vi "Teleop.vi"(10 "Match Info":T1={"Autonomous Elapsed Seconds"=0.0, "TeleOp Elapsed Seconds"=0.0, "Disabled Elapsed Seconds"=0.0, "Visited Autonomous"=FALSE, "Visited TeleOp"=FALSE, "Visited Disabled"=FALSE, "Autonomous Settings"={"Autonomous Style"=enum."Independent", "VI Refnum"=refnum}}, 11 "Call Context":T2) -> ()   [LabVIEW 2013]
doc: "This VI is called for each TeleOp packet received from the DS where the robot is not disabled. It is often used to read from the joysticks and update I/O or to update setpoints for timed control loops. It should complete and return within 20 milliseconds or it may miss DS packets."
uses:
  <vilib>/Rock Robotics/WPI/DriverStation/WPI_DriverStationDerivedRobotMode.ctl
  <vilib>/Rock Robotics/WPI/DriverStation/WPI_DriverStationMatch Info.ctl
  <vilib>/Rock Robotics/WPI/DriverStation/DriverStationLCD/WPI_DriverStationLCDLCDLine.ctl
  Robot Global Data.vi
  <vilib>/Rock Robotics/WPI/Joystick/WPI_JoystickGetSetRefNum.vi
  <vilib>/Rock Robotics/WPI/RobotDrive/WPI_RobotDriveGetSetRefNum.vi
  <vilib>/Rock Robotics/WPI/Solenoid/WPI_SolenoidSetEnum.vi
  <vilib>/Rock Robotics/WPI/Solenoid/WPI_SolenoidValue.ctl
panel:
  out "Numeric 1":dbl(slide) scale=0.0..100.0
  out "Boolean 2":bool
  out "Boolean 1":bool
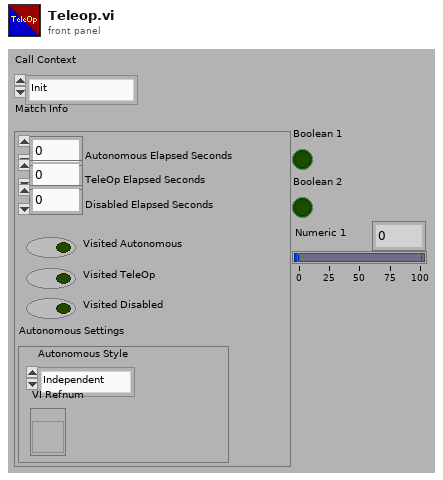
[diagram p1: front panel]
types:
  T1 = typedef "WPI_DriverStationMatch Info.ctl" = cluster{"Autonomous Elapsed Seconds":dbl, "TeleOp Elapsed Seconds":dbl, "Disabled Elapsed Seconds":dbl, "Visited Autonomous":bool, "Visited TeleOp":bool, "Visited Disabled":bool, "Autonomous Settings":cluster{"Autonomous Style":enum16{"Iterative", "Independent"}, "VI Refnum":refnum<vi>}}
  T2 = typedef "WPI_DriverStationDerivedRobotMode.ctl" = enum16{"Init", "Execute", "Stop"}
  T3 = typedef "WPI_DriverStationLCDLCDLine.ctl" = enum16{"Main - Line 1", "User - Line 2", "User - Line 3", "User - Line 4", "User - Line 5", "User - Line 6"}
  T4 = typedef "WPI_JoystickDevRef.ctl" = cluster{"Device":T5}
  T5 = typedef "WPI_JoystickDeviceEnum.ctl" = enum16{"USB 1", "USB 2", "USB 3", "USB 4", "Kinect 1", "Kinect 2"}
  T6 = typedef "WPI_JoystickButtonState.ctl" = cluster{"Button 1":bool, "Button 2":bool, "Button 3":bool, "Button 4":bool, "Button 5":bool, "Button 6":bool, "Button 7":bool, "Button 8":bool, "Button 9":bool, "Button 10":bool, "Button 11":bool, "Button 12":bool}
  T7 = cluster{"axis 1 (x)":dbl, "axis 2 (y)":dbl, "axis 3 (throttle)":dbl, "axis 4":dbl, "axis 5":dbl, "axis 6":dbl}
  T8 = typedef "WPI_SolenoidValue.ctl" = enum16{"Off", "On", "Forward", "Reverse"}
  T9 = typedef "WPI_SolenoidDevRef.ctl" = cluster{"DevStatus":errorcluster, "Solenoid Module":T10, "Forward Solenoid Channel":T11, "Reverse Solenoid Channel":T11}
  T10 = typedef "FPGA_TypedefSolenoidModule.ctl" = enum16{"Solenoid Module 1", "Solenoid Module 2"}
  T11 = typedef "WPI_SolenoidChannel.ctl" = enum8{"Solenoid 1", "Solenoid 2", "Solenoid 3", "Solenoid 4", "Solenoid 5", "Solenoid 6", "Solenoid 7", "Solenoid 8", "Invalid"}
  T12 = typedef "WPI_RobotDriveDevRef.ctl" = cluster{"DevStatus":errorcluster, "Motors[]":T13[], "Square Inputs":bool, "Max Output":dbl, "Isochronous":bool}
  T13 = typedef "WPI_MotorControlDeviceRef.ctl" = cluster{"DeviceStatus":errorcluster, "Type":enum16{"PWM", "CAN"}, "PWM":cluster{"Digital Module":T14, "PWM Channel":T15, "DeadBand":T16}, "CAN":cluster{"Device Number":u8, "Control Mode":T17, "Semaphore":T18, "Max Vout":dbl}, "Invert":bool, "TransformRef":T19, "InvTransformRef":T19}
  T14 = typedef "FPGA_TypedefDigitalModule.ctl" = enum16{"Digital Module 1", "Digital Module 2"}
  T15 = typedef "FPGA_DIOPWMChannel.ctl" = enum8{"PWM 1", "PWM 2", "PWM 3", "PWM 4", "PWM 5", "PWM 6", "PWM 7", "PWM 8", "PWM 9", "PWM 10", "Invalid"}
  T16 = typedef "WPI_PWMDeadband.ctl" = cluster{"Name":string, "maxPositivePwm":i32, "minPositivePwm":i32, "centerPwm":i32, "maxNegativePwm":i32, "minNegativePwm":i32, "angularRange":u16}
  T17 = typedef "WPI_CANJaguar_ControlMode.ctl" = enum8{"Percent VBus", "Current", "Speed", "Position", "Voltage"}
  T18 = typedef "Semaphore RefNum" = refnum<k1>
  T19 = typedef "WPI_PWMTransform_ConPane.ctl" = refnum<vi>
  T20 = enum16{"Start", "Reset", "Reset 2", "Reset Delay", "Reset 3", "Manual", "Wait for Firing Latch", "Get ready to Fire", "Disengage Gearbox", "Ready to Fire", "Firing", "Firing Completed", "Reengage Gearbox"}
  T21 = typedef "WPI_DigitalInputDevRef.ctl" = cluster{"DevStatus":errorcluster, "DIO Channel":T22, "Digital Module":T14}
  T22 = typedef "FPGA_DIOChannel.ctl" = enum8{"DIO 1", "DIO 2", "DIO 3", "DIO 4", "DIO 5", "DIO 6", "DIO 7", "DIO 8", "DIO 9", "DIO 10", "DIO 11", "DIO 12", "DIO 13", "DIO 14", "Invalid"}
  T23 = typedef "WPI_ServoDeviceRef.ctl" = cluster{"DeviceStatus":errorcluster, "Digital Module":T14, "PWM Channel":T15, "DeadBand":T16}
  T24 = typedef "WPI_AnalogChannelDevRef.ctl" = cluster{"DevStatus":errorcluster, "Analog Module":T25, "Analog Channel":T26}
  T25 = typedef "FPGA_TypedefAnalogModule.ctl" = enum16{"Analog Module 1", "Analog Module 2"}
  T26 = typedef "FPGA_AIChannel.ctl" = enum8{"AI 1", "AI 2", "AI 3", "AI 4", "AI 5", "AI 6", "AI 7", "AI 8", "Invalid"}
  T27 = typedef "WPI_RelayDevRef.ctl" = cluster{"DevStatus":errorcluster, "Relay Channel":T28, "Digital Module":T14, "Relay Direction":T29}
  T28 = typedef "FPGA_DIORelayChannel.ctl" = enum8{"Relay 1", "Relay 2", "Relay 3", "Relay 4", "Relay 5", "Relay 6", "Relay 7", "Relay 8", "Invalid"}
  T29 = typedef "WPI_RelayDirection.ctl" = enum16{"Both directions", "Forward only", "Reverse only"}
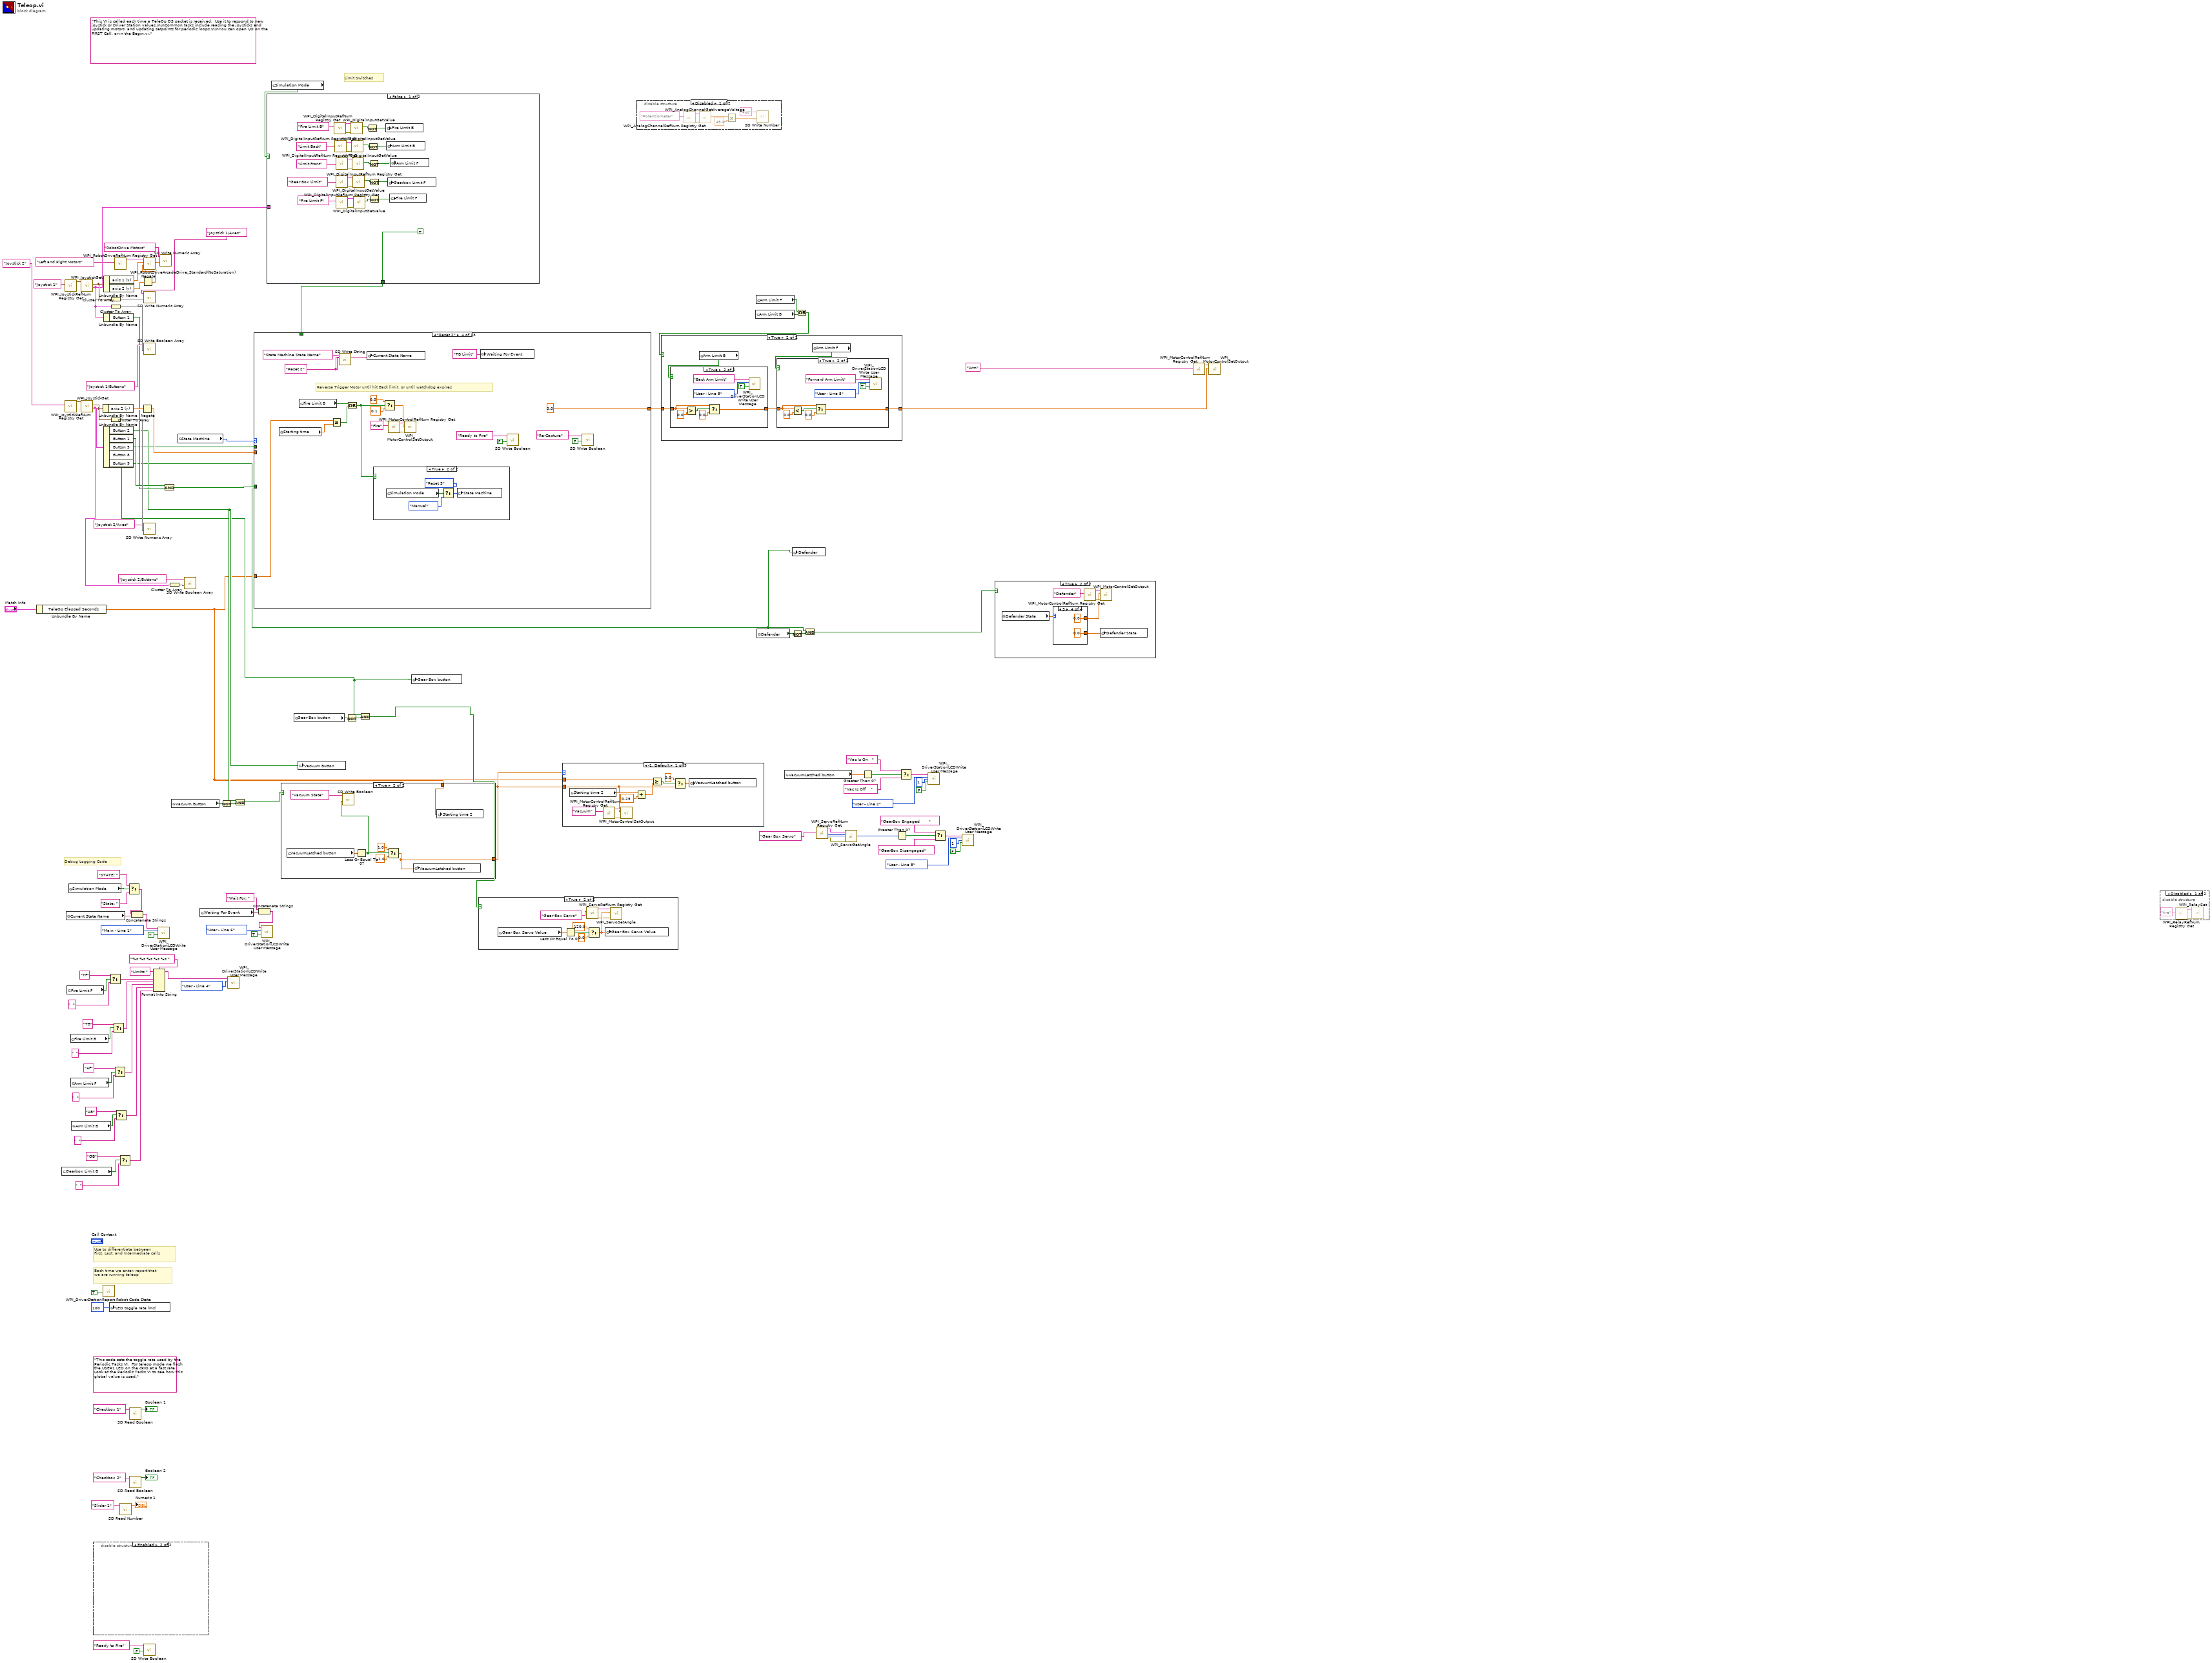
[diagram p0: block diagram]
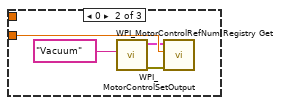
[diagram p2: hidden frame]
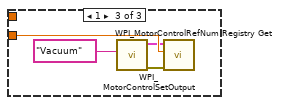
[diagram p3: hidden frame]
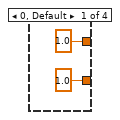
[diagram p6: hidden frame]
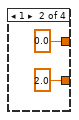
[diagram p7: hidden frame]
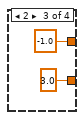
[diagram p8: hidden frame]
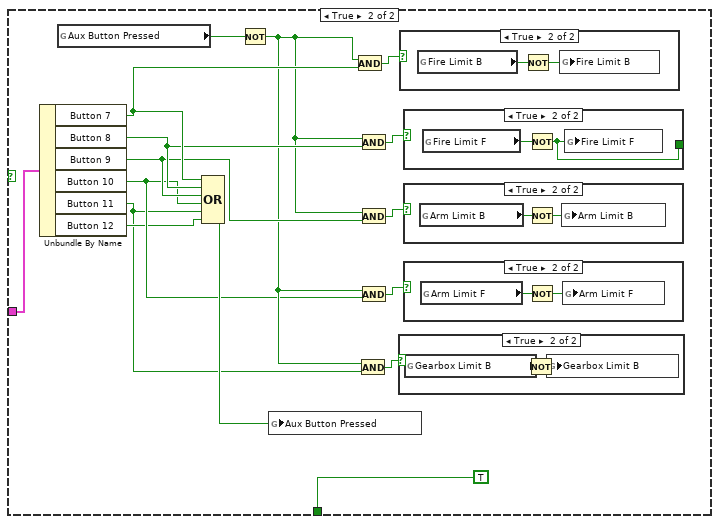
[diagram p9: hidden frame]
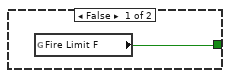
[diagram p13: hidden frame]
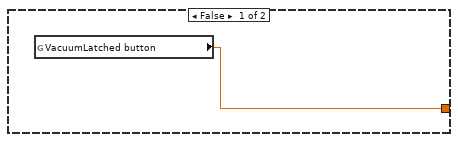
[diagram p15: hidden frame]
diagram:
  (unwired) "This code sets the toggle rate used by the Periodic Tasks VI.  For teleop mode we flash the USER1 LED on the cRIO at a fast rate.  Look at the Periodic Tasks VI to see how this global value is used."
  (unwired) "This VI is called each time a TeleOp DS packet is received.  Use it to respond to new joystick or Driver Station values.\n\nCommon tasks include reading the joysticks and updating motors, and updating setpoints for periodic loops.\n\nYou can open I/O on the FIRST Call, or in the Begin.vi."
  # "Limit Switches"
  # "Debug Logging Code"
  # "Each time we enter, report that\nwe are running teleop"
  # "Use to differentiate between\nFirst, Last, and Intermediate calls"
  n1 = Unbundle By Name("Match Info") -> ("TeleOp Elapsed Seconds"=w1:dbl)
  n2 = global read "Robot Global Data.vi" "Gearbox Limit B"() -> (w36:bool)
  n3 = call <vilib>:"WPI_JoystickRefNum Registry Get.vi"("refnum name"="Joystick 1") -> ("JoystickDevRef"=w115:T4)  [unwired: 1 in, 9 out]
  n4 = call <vilib>:"WPI_JoystickRefNum Registry Get.vi"("refnum name"="Joystick 2") -> ("JoystickDevRef"=w98:T4)  [unwired: 1 in, 9 out]
  n5 = global read "Robot Global Data.vi" "Current State Name"() -> (w63:string)
  n6 = global read "Robot Global Data.vi" "Fire Limit F"() -> (w40:bool)
  n7 = global read "Robot Global Data.vi" "Simulation Mode"() -> (w29:bool)
  n8 = global read "Robot Global Data.vi" "Fire Limit B"() -> (w39:bool)
  n9 = global read "Robot Global Data.vi" "Arm Limit F"() -> (w38:bool)
  n10 = global read "Robot Global Data.vi" "Arm Limit B"() -> (w37:bool)
  n11 = call <vilib>:"WPI_JoystickGet.vi"("JoystickDevRef"=w115) -> ("Buttons"=w25:T6, "Axes"=w110:T7)  [unwired: 1 in, 4 out]
  n12 = call <vilib>:"WPI_JoystickGet.vi"("JoystickDevRef"=w98) -> ("Buttons"=w92:T6, "Axes"=w95:T7)  [unwired: 1 in, 4 out]
  n13 = disable-structure shown="Enabled" {
    frame Disabled {
      n14 = case shown="True" {
        selector: _ -> [_ _]
        frame False {
          n15 = call <vilib>:"WPI_SolenoidRefNum Registry Get.vi"("refnum name"="Gear Box Clutch") -> ("error out"=w126:errorcluster, "SolenoidDevRef"=w127:T9)  [unwired: 9 in]
          n16 = call-poly <vilib>:"WPI_SolenoidSet.vi"("error in (no error)"=w126, "Value"=WPI_SolenoidValue."Off", "SolenoidDevRef"=w127) -> ()  [unwired: 7 in, 2 out]
          n17 = call <vilib>:"WPI_DriverStationLCDWrite User Message.vi"("line text"="Gear Box Clutch off", "line"=WPI_DriverStationLCDLCDLine."User - Line 2", "starting column"=i8 1, "clear line before write (T)"=FALSE) -> ()  [unwired: 11 in, 1 out]
        }
        frame True {
          n18 = call <vilib>:"WPI_SolenoidRefNum Registry Get.vi"("refnum name"="Gear Box Clutch") -> ("error out"=w134:errorcluster, "SolenoidDevRef"=w135:T9)  [unwired: 9 in]
          n19 = call-poly <vilib>:"WPI_SolenoidSet.vi"("error in (no error)"=w134, "Value"=WPI_SolenoidValue."Forward", "SolenoidDevRef"=w135) -> ()  [unwired: 7 in, 2 out]
          n20 = call <vilib>:"WPI_DriverStationLCDWrite User Message.vi"("line text"="Gear Box Clutch off", "line"=WPI_DriverStationLCDLCDLine."User - Line 2", "starting column"=i8 1, "clear line before write (T)"=FALSE) -> ()  [unwired: 11 in, 1 out]
        }
      }
    }
    frame Enabled {
    }
  }
  n21 = Unbundle By Name(w95) -> ("axis 2 (y)"=w91:dbl)
  n22 = call <vilib>:"WPI_DriverStationReport Robot Code State.vi"("TeleOp"=TRUE ("Autonomous")) -> ()  [unwired: 10 in, 1 out]
  n23 = Unbundle By Name(w110) -> ("axis 1 (x)"=w117:dbl, "axis 2 (y)"=w58:dbl)
  n24 = Unbundle By Name(w25) -> ("Button 1"=w89:bool)
  n25 = Unbundle By Name(w92) -> ("Button 2"=w80:bool, "Button 1"=w90:bool, "Button 5"=w66:bool, "Button 8"=w19:bool, "Button 9"=w18:bool)
  n26 = Select(t="TF", s=w40, f="  ") -> (s? t:f=w46:string)
  n27 = global write "Robot Global Data.vi" "LED toggle rate (ms)"(u32 100 ("LED ms toggle rate")) -> ()
  n28 = Cluster To Array(cluster=w110) -> (array=w109:dbl[])
  n29 = Cluster To Array(cluster=w25) -> (array=w112:bool[])
  n30 = Cluster To Array(cluster=w95) -> (array=w94:dbl[])
  n31 = Select(t="TB", s=w39, f="  ") -> (s? t:f=w45:string)
  n32 = Select(t="AF", s=w38, f="  ") -> (s? t:f=w44:string)
  n33 = call <vilib>:"WPI_RobotDriveRefNum Registry Get.vi"("refnum name"="Left and Right Motors") -> ("RobotDriveDevRef"=w118:T12)  [unwired: 1 in, 9 out]
  n34 = Select(t="AB", s=w37, f="  ") -> (s? t:f=w43:string)
  n35 = Select(t="GB", s=w36, f="  ") -> (s? t:f=w42:string)
  n36 = call <vilib>:"SD Read Number.vi"("Name"="Slider 1" ("refnum name")) -> ("Numeric"=→"Numeric 1":dbl)  [unwired: 8 in, 2 out]
  n37 = Select(t="STATE: " ("line text"), s=w29, f="State: " ("line text")) -> (s? t:f=w26:string)
  n38 = call <vilib>:"SD Read Boolean.vi"("Name"="Checkbox 1" ("refnum name")) -> ("Boolean"=→"Boolean 1":bool)  [unwired: 8 in, 2 out]
  n39 = call <vilib>:"SD Read Boolean.vi"("Name"="Checkbox 2" ("refnum name")) -> ("Boolean"=→"Boolean 2":bool)  [unwired: 8 in, 2 out]
  n40 = Concatenate Strings(w26, w63) -> (w62:string)
  n41 = Negate(x=w91) -> (-x=w83:dbl)
  n42 = Negate(x=w58) -> (-x=w57:dbl)
  n43 = call <vilib>:"SD Write Boolean.vi"("Boolean"=FALSE, "Name"="Ready to Fire") -> ()  [unwired: 8 in, 2 out]
  n44 = call <vilib>:"WPI_RobotDriveArcadeDrive_Standard(NoSaturation).vi"("Y axis value"=w57, "X axis value"=w117, "RobotDriveDevRef"=w118) -> ("Motor Values"=w106:dbl[])  [unwired: 1 in, 7 out]
  n45 = call <vilib>:"SD Write Numeric Array.vi"("Numeric Array"=w109, "Name"="Joystick 1/Axes") -> ()  [unwired: 8 in, 2 out]
  n46 = call <vilib>:"SD Write Boolean Array.vi"("Boolean Array"=w112, "Name"="Joystick 1/Buttons") -> ()  [unwired: 8 in, 2 out]
  n47 = call <vilib>:"SD Write Numeric Array.vi"("Numeric Array"=w94, "Name"="Joystick 2/Axes") -> ()  [unwired: 8 in, 2 out]
  n48 = Format Into String(format string="%s %s %s %s %s " ("initial string"), initial string="Limits ", w46, w45, w44, w43, w42) -> (resulting string=w41:string)  [unwired: 1 in, 1 out]
  n49 = call <vilib>:"WPI_DriverStationLCDWrite User Message.vi"("line text"=w62, "line"=WPI_DriverStationLCDLCDLine."Main - Line 1", "clear line before write (T)"=TRUE) -> ()  [unwired: 12 in, 1 out]
  n50 = call <vilib>:"SD Write Numeric Array.vi"("Numeric Array"=w106, "Name"="RobotDrive Motors") -> ()  [unwired: 8 in, 2 out]
  n51 = And(x=w90, y=w89) -> (x .and. y?=w78:bool)
  n52 = Cluster To Array(cluster=w92) -> (array=w97:bool[])
  n53 = global read "Robot Global Data.vi" "Vacuum Button"() -> (w81:bool)
  n54 = global read "Robot Global Data.vi" "State Machine"() -> (w79:T20)
  n55 = call <vilib>:"SD Write Boolean Array.vi"("Boolean Array"=w97, "Name"="Joystick 2/Buttons") -> ()  [unwired: 8 in, 2 out]
  n56 = global read "Robot Global Data.vi" "Waiting For Event"() -> (w22:string)
  n57 = Not(x=w81) -> (.not. x?=w82:bool)
  n58 = call <vilib>:"WPI_DriverStationLCDWrite User Message.vi"("line text"=w41, "line"=WPI_DriverStationLCDLCDLine."User - Line 4") -> ()  [unwired: 13 in, 1 out]
  n59 = And(x=w80, y=w82) -> (x .and. y?=w76:bool)
  n60 = Concatenate Strings("Wait For: " ("string"), w22) -> (w20:string)
  n61 = call <vilib>:"WPI_DriverStationLCDWrite User Message.vi"("line text"=w20, "line"=WPI_DriverStationLCDLCDLine."User - Line 6", "clear line before write (T)"=TRUE) -> ()  [unwired: 12 in, 1 out]
  n62 = global read "Robot Global Data.vi" "Simulation Mode"() -> (w35:bool)
  n63 = case shown="False" w35 {
    tunnel: [TRUE TRUE] -> w32
    tunnel: w25 -> [_ w178]
    frame False {
      n64 = call <vilib>:"WPI_DigitalInputRefNum Registry Get.vi"("refnum name"="Fire Limit B") -> ("error out"=w158:errorcluster, "DigitalInputDevRef"=w157:T21)  [unwired: 9 in]
      n65 = call <vilib>:"WPI_DigitalInputRefNum Registry Get.vi"("refnum name"="Limit Back") -> ("error out"=w154:errorcluster, "DigitalInputDevRef"=w153:T21)  [unwired: 9 in]
      n66 = call <vilib>:"WPI_DigitalInputRefNum Registry Get.vi"("refnum name"="Limit Front") -> ("error out"=w151:errorcluster, "DigitalInputDevRef"=w150:T21)  [unwired: 9 in]
      n67 = call <vilib>:"WPI_DigitalInputRefNum Registry Get.vi"("refnum name"="Fire Limit F") -> ("error out"=w161:errorcluster, "DigitalInputDevRef"=w162:T21)  [unwired: 9 in]
      n68 = call <vilib>:"WPI_DigitalInputRefNum Registry Get.vi"("refnum name"="Gear Box Limit") -> ("error out"=w147:errorcluster, "DigitalInputDevRef"=w146:T21)  [unwired: 9 in]
      n69 = call <vilib>:"WPI_DigitalInputGetValue.vi"("error in (no error)"=w158, "DigitalInputDevRef"=w157) -> ("Value"=w155:bool)  [unwired: 7 in, 2 out]
      n70 = call <vilib>:"WPI_DigitalInputGetValue.vi"("error in (no error)"=w154, "DigitalInputDevRef"=w153) -> ("Value"=w140:bool)  [unwired: 7 in, 2 out]
      n71 = call <vilib>:"WPI_DigitalInputGetValue.vi"("error in (no error)"=w151, "DigitalInputDevRef"=w150) -> ("Value"=w149:bool)  [unwired: 7 in, 2 out]
      n72 = call <vilib>:"WPI_DigitalInputGetValue.vi"("error in (no error)"=w147, "DigitalInputDevRef"=w146) -> ("Value"=w145:bool)  [unwired: 7 in, 2 out]
      n73 = call <vilib>:"WPI_DigitalInputGetValue.vi"("error in (no error)"=w161, "DigitalInputDevRef"=w162) -> ("Value"=w159:bool)  [unwired: 7 in, 2 out]
      n74 = Not(x=w155) -> (.not. x?=w139:bool)
      n75 = Not(x=w140) -> (.not. x?=w143:bool)
      n76 = Not(x=w149) -> (.not. x?=w142:bool)
      n77 = Not(x=w145) -> (.not. x?=w141:bool)
      n78 = Not(x=w159) -> (.not. x?=w138:bool)
      n79 = global write "Robot Global Data.vi" "Fire Limit B"(w139) -> ()
      n80 = global write "Robot Global Data.vi" "Arm Limit B"(w143) -> ()
      n81 = global write "Robot Global Data.vi" "Gearbox Limit F"(w141) -> ()
      n82 = global write "Robot Global Data.vi" "Fire Limit F"(w138) -> ()
      n83 = global write "Robot Global Data.vi" "Arm Limit F"(w142) -> ()
    }
    frame True {
      n84 = Unbundle By Name(w178) -> ("Button 7"=w176:bool, "Button 8"=w169:bool, "Button 9"=w168:bool, "Button 10"=w166:bool, "Button 11"=w164:bool, "Button 12"=w165:bool)
      n85 = global read "Robot Global Data.vi" "Aux Button Pressed"() -> (w177:bool)
      n86 = Compound Arithmetic op=OR(w176, w169, w168, w166, w164, w165) -> (w175:bool)
      n87 = Not(x=w177) -> (.not. x?=w167:bool)
      n88 = global write "Robot Global Data.vi" "Aux Button Pressed"(w175) -> ()
      n89 = And(x=w167, y=w176) -> (x .and. y?=w174:bool)
      n90 = And(x=w167, y=w164) -> (x .and. y?=w170:bool)
      n91 = And(x=w167, y=w169) -> (x .and. y?=w173:bool)
      n92 = And(x=w167, y=w168) -> (x .and. y?=w172:bool)
      n93 = And(x=w167, y=w166) -> (x .and. y?=w171:bool)
      n94 = case shown="True" w170 {
        frame False {
        }
        frame True {
          n95 = global read "Robot Global Data.vi" "Gearbox Limit B"() -> (w180:bool)
          n96 = Not(x=w180) -> (.not. x?=w179:bool)
          n97 = global write "Robot Global Data.vi" "Gearbox Limit B"(w179) -> ()
        }
      }
      n98 = case shown="True" w174 {
        frame False {
        }
        frame True {
          n99 = global read "Robot Global Data.vi" "Fire Limit B"() -> (w189:bool)
          n100 = Not(x=w189) -> (.not. x?=w188:bool)
          n101 = global write "Robot Global Data.vi" "Fire Limit B"(w188) -> ()
        }
      }
      n102 = case shown="True" w173 {
        tunnel: [w185 w186] -> _
        frame False {
          n103 = global read "Robot Global Data.vi" "Fire Limit F"() -> (w185:bool)
        }
        frame True {
          n104 = global read "Robot Global Data.vi" "Fire Limit F"() -> (w187:bool)
          n105 = Not(x=w187) -> (.not. x?=w186:bool)
          n106 = global write "Robot Global Data.vi" "Fire Limit F"(w186) -> ()
        }
      }
      n107 = case shown="True" w172 {
        frame False {
        }
        frame True {
          n108 = global read "Robot Global Data.vi" "Arm Limit B"() -> (w184:bool)
          n109 = Not(x=w184) -> (.not. x?=w183:bool)
          n110 = global write "Robot Global Data.vi" "Arm Limit B"(w183) -> ()
        }
      }
      n111 = case shown="True" w171 {
        frame False {
        }
        frame True {
          n112 = global read "Robot Global Data.vi" "Arm Limit F"() -> (w182:bool)
          n113 = Not(x=w182) -> (.not. x?=w181:bool)
          n114 = global write "Robot Global Data.vi" "Arm Limit F"(w181) -> ()
        }
      }
    }
  }
  n115 = case shown="\"Reset 2\"" w79 {
    selector: w79 -> [_ _ w225 _ w252 _ _ _ _ _ w348 _ _]
    tunnel: w83 -> [_ _ _ _ w258 w262 w281 w282 w302 w315 w335 w367 w374]
    tunnel: [0.0 w201 0.0 0.0 w258 w262 w281 w283 w302 w315 w335 w367 w374] -> w77
    tunnel: w78 -> [_ _ _ _ _ _ _ _ _ w311 _ _ _]
    tunnel: w1 -> [w191 w210 w220 w235 _ _ w278 w284 w297 w308 w333 w357 w368]
    tunnel: w66 -> [_ _ _ _ _ w261 _ _ _ _ _ _ _]
    tunnel: w32 -> [_ _ _ _ _ _ _ _ _ _ _ _ _]
    frame "Start" {
      w198 = "Start" ("line text")
      # "Set watchdog timer for Trigger motor set"
      n116 = global read "Robot Global Data.vi" "Simulation Mode"() -> (w195:bool)
      n117 = global write "Robot Global Data.vi" "State Machine"(T20."Reset 2" ("State Machine")) -> ()
      n118 = call <vilib>:"SD Write String.vi"("Table Prefix"=w198, "Name"="State Machine State Name") -> ()  [unwired: 8 in, 2 out]
      n119 = Select(t=10.0 ("y"), s=w195, f=3.0 ("y")) -> (s? t:f=w192:dbl)
      n120 = global write "Robot Global Data.vi" "Current State Name"(w198) -> ()
      n121 = Add(x=w191, y=w192) -> (x+y=w196:dbl)
      n122 = global write "Robot Global Data.vi" "Starting time"(w196) -> ()
      n123 = global write "Robot Global Data.vi" "Waiting For Event"("Auto" ("Waiting For Event")) -> ()
    }
    frame "Reset" {
      w211 = "Reset" ("line text")
      # "Set watchdog timer for Trigger motor set"
      # "Pull Arm back until hit Back limit\nthen turn power off"
      n124 = global read "Robot Global Data.vi" "Arm Limit B"() -> (w206:bool)
      n125 = Add(x=w210, y=1.0) -> (x+y=w208:dbl)
      n126 = global write "Robot Global Data.vi" "Starting time"(w208) -> ()
      n127 = case shown="True" w206 {
        frame False {
        }
        frame True {
          n128 = global write "Robot Global Data.vi" "State Machine"(T20."Reset Delay" ("State Machine")) -> ()
        }
      }
      n129 = call <vilib>:"SD Write String.vi"("Table Prefix"=w211, "Name"="State Machine State Name") -> ()  [unwired: 8 in, 2 out]
      n130 = global write "Robot Global Data.vi" "Current State Name"(w211) -> ()
      n131 = global write "Robot Global Data.vi" "Waiting For Event"("AB Limit" ("Waiting For Event")) -> ()
      n132 = call <vilib>:"SD Write Boolean.vi"("Boolean"=FALSE, "Name"="Ready to Fire") -> ()  [unwired: 8 in, 2 out]
      n133 = call <vilib>:"WPI_MotorControlRefNum Registry Get.vi"("refnum name"="Fire") -> ("error out"=w202:errorcluster, "MotorControlDevRef"=w205:T13)  [unwired: 9 in]
      n134 = Select(t=0.0, s=w206, f=0.0) -> (s? t:f=w201:dbl)
      n135 = call <vilib>:"WPI_MotorControlSetOutput.vi"("error in (no error)"=w202, "Output"=-0.2, "MotorControlDevRef"=w205) -> ()  [unwired: 6 in, 3 out]
    }
    frame "Reset Delay" {
      n136 = global read "Robot Global Data.vi" "Starting time"() -> (w222:dbl)
      n137 = Greater Or Equal?(x=w220, y=w222) -> (x >= y?=w223:bool)
      n138 = Select(t=T20."Reset 2" ("State Machine"), s=w223, f=w225) -> (s? t:f=w224:T20)
      n139 = Add(x=w220, y=3.0 ("x")) -> (x+y=w219:dbl)
      n140 = Select(t=w219, s=w223, f=w222) -> (s? t:f=w218:dbl)
      n141 = global write "Robot Global Data.vi" "State Machine"(w224) -> ()
      n142 = global write "Robot Global Data.vi" "Starting time"(w218) -> ()
    }
    frame "Reset 2" {
      w236 = "Reset 2" ("line text")
      # "Reverse Trigger Motor until hit Back limit, or until watchdog expires"
      n143 = global read "Robot Global Data.vi" "Starting time"() -> (w234:dbl)
      n144 = global read "Robot Global Data.vi" "Fire Limit B"() -> (w231:bool)
      n145 = Greater Or Equal?(x=w235, y=w234) -> (x >= y?=w233:bool)
      n146 = call <vilib>:"SD Write String.vi"("Table Prefix"=w236, "Name"="State Machine State Name") -> ()  [unwired: 8 in, 2 out]
      n147 = Or(x=w231, y=w233) -> (x .or. y?=w230:bool)
      n148 = global write "Robot Global Data.vi" "Current State Name"(w236) -> ()
      n149 = case shown="True" w230 {
        frame False {
        }
        frame True {
          n150 = global read "Robot Global Data.vi" "Simulation Mode"() -> (w250:bool)
          n151 = Select(t=T20."Reset 3" ("State Machine"), s=w250, f=T20."Manual" ("State Machine")) -> (s? t:f=w247:T20)
          n152 = global write "Robot Global Data.vi" "State Machine"(w247) -> ()
        }
      }
      n153 = Select(t=0.0, s=w230, f=0.1) -> (s? t:f=w238:dbl)
      n154 = call <vilib>:"WPI_MotorControlRefNum Registry Get.vi"("refnum name"="Fire") -> ("error out"=w244:errorcluster, "MotorControlDevRef"=w243:T13)  [unwired: 9 in]
      n155 = call <vilib>:"WPI_MotorControlSetOutput.vi"("error in (no error)"=w244, "Output"=w238, "MotorControlDevRef"=w243) -> ()  [unwired: 6 in, 3 out]
      n156 = global write "Robot Global Data.vi" "Waiting For Event"("TB Limit" ("Waiting For Event")) -> ()
      n157 = call <vilib>:"SD Write Boolean.vi"("Boolean"=FALSE, "Name"="Ready to Fire") -> ()  [unwired: 8 in, 2 out]
      n158 = call <vilib>:"SD Write Boolean.vi"("Boolean"=FALSE, "Name"="Re-Capture") -> ()  [unwired: 8 in, 2 out]
    }
    frame "Reset 3" {
      w256 = "Reset 3" ("line text")
      # "Wait until Arm Back limit switch is off"
      n159 = call <vilib>:"SD Write String.vi"("Table Prefix"=w256, "Name"="State Machine State Name") -> ()  [unwired: 8 in, 2 out]
      n160 = global read "Robot Global Data.vi" "Arm Limit B"() -> (w254:bool)
      n161 = global write "Robot Global Data.vi" "Current State Name"(w256) -> ()
      n162 = Select(t=w252, s=w254, f=T20."Manual" ("s? t:f")) -> (s? t:f=w253:T20)
      n163 = global write "Robot Global Data.vi" "State Machine"(w253) -> ()
      n164 = global write "Robot Global Data.vi" "Waiting For Event"("AB Limit Off" ("Waiting For Event")) -> ()
    }
    frame "Manual", Default {
      w263 = "Manual" ("line text")
      # "If hit rear Arm limit switch, get ready to fire, \nelse if Reset button hit, start reset"
      n165 = global read "Robot Global Data.vi" "Arm Limit B"() -> (w260:bool)
      n166 = Or(x=w260, y=w261) -> (x .or. y?=w264:bool)
      n167 = case shown="True" w264 {
        tunnel: w260 -> [_ w276]
        frame False {
        }
        frame True {
          n168 = Select(t="Reason: Limit Back hit" ("line text"), s=w276, f="Reason Button 5 pressed:" ("line text")) -> (s? t:f=w271:string)
          n169 = Select(t=T20."Wait for Firing Latch" ("State Machine"), s=w276, f=T20."Reset") -> (s? t:f=w269:T20)
          n170 = call <vilib>:"WPI_DriverStationLCDWrite User Message.vi"("line text"=w271, "line"=WPI_DriverStationLCDLCDLine."User - Line 3", "clear line before write (T)"=TRUE) -> ()  [unwired: 12 in, 1 out]
          n171 = global write "Robot Global Data.vi" "State Machine"(w269) -> ()
        }
      }
      n172 = call <vilib>:"SD Write String.vi"("Table Prefix"=w263, "Name"="State Machine State Name") -> ()  [unwired: 8 in, 2 out]
      n173 = global write "Robot Global Data.vi" "Current State Name"(w263) -> ()
      n174 = global write "Robot Global Data.vi" "Waiting For Event"("AB Limit | Btn 5" ("Waiting For Event")) -> ()
      n175 = call <vilib>:"SD Write Boolean.vi"("Boolean"=FALSE, "Name"="Ready to Fire") -> ()  [unwired: 8 in, 2 out]
    }
    frame "Wait for Firing Latch" {
      # "Wait .5 secs before turning off arm power to give time for arm latch to engage"
      n176 = Add(x=0.5 ("Starting time"), y=w278) -> (x+y=w279:dbl)
      n177 = global write "Robot Global Data.vi" "Starting time"(w279) -> ()
      n178 = global write "Robot Global Data.vi" "State Machine"(T20."Get ready to Fire" ("State Machine")) -> ()
    }
    frame "Get ready to Fire" {
      w288 = "Get ready to Fire" ("line text")
      # "After latch has time to engage, prepare to disengage gearbox"
      n179 = global read "Robot Global Data.vi" "Starting time"() -> (w286:dbl)
      n180 = Greater Or Equal?(x=w284, y=w286) -> (x >= y?=w285:bool)
      n181 = call <vilib>:"SD Write String.vi"("Table Prefix"=w288, "Name"="State Machine State Name") -> ()  [unwired: 8 in, 2 out]
      n182 = case shown="True" w285 {
        tunnel: w284 -> [_ w293]
        tunnel: [w290 0.0] -> w283
        tunnel: w282 -> [w290 _]
        frame False {
        }
        frame True {
          # "Turn Off Arm Motor"
          # "Wait .5 secs before disengaging gearbox to give time for arm latch to engage"
          n183 = Add(x=0.5 ("Starting time"), y=w293) -> (x+y=w294:dbl)
          n184 = global write "Robot Global Data.vi" "Starting time"(w294) -> ()
          n185 = global write "Robot Global Data.vi" "State Machine"(T20."Disengage Gearbox" ("State Machine")) -> ()
        }
      }
      n186 = global write "Robot Global Data.vi" "Current State Name"(w288) -> ()
      n187 = global write "Robot Global Data.vi" "Waiting For Event"("Auto" ("Waiting For Event")) -> ()
    }
    frame "Disengage Gearbox" {
      w300 = "Disengage Gearbox" ("line text")
      # "After delay, disengage gearbox"
      n188 = global read "Robot Global Data.vi" "Starting time"() -> (w299:dbl)
      n189 = Greater Or Equal?(x=w297, y=w299) -> (x >= y?=w298:bool)
      n190 = call <vilib>:"SD Write String.vi"("Table Prefix"=w300, "Name"="State Machine State Name") -> ()  [unwired: 8 in, 2 out]
      n191 = case shown="True" w298 {
        frame False {
        }
        frame True {
          n192 = call <vilib>:"WPI_ServoRefNum Registry Get.vi"("refnum name"="Gear Box Servo") -> ("error out"=w304:errorcluster, "ServoDeviceRef"=w305:T23)  [unwired: 9 in]
          n193 = global write "Robot Global Data.vi" "State Machine"(T20."Ready to Fire" ("State Machine")) -> ()
          n194 = call <vilib>:"WPI_ServoSetAngle.vi"("error in (no error)"=w304, "Angle"=0, "ServoDeviceRef"=w305) -> ()  [unwired: 7 in, 2 out]
        }
      }
      n195 = global write "Robot Global Data.vi" "Current State Name"(w300) -> ()
      n196 = global write "Robot Global Data.vi" "Waiting For Event"("Timer" ("Waiting For Event")) -> ()
    }
    frame "Ready to Fire" {
      w310 = "Ready to fire" ("line text")
      # "If both trigger btns pressed and vacuum is off\nthen fire"
      n197 = call <vilib>:"SD Write Boolean.vi"("Boolean"=TRUE, "Name"="Ready to Fire") -> ()  [unwired: 8 in, 2 out]
      n198 = call <vilib>:"SD Write String.vi"("Table Prefix"=w310, "Name"="State Machine State Name") -> ()  [unwired: 8 in, 2 out]
      n199 = case shown="True" w311 {
        tunnel: w308 -> [_ w316]
        frame False {
        }
        frame True {
          n200 = global read "Robot Global Data.vi" "VacuumLatched button"() -> (w317:dbl)
          n201 = case shown="0, Default" w317 {
            tunnel: w316 -> [w319 _]
            frame 0, Default {
              # "Set watchdog timer in case never hit limit switch"
              n202 = Add(x=3.0 ("Starting time"), y=w319) -> (x+y=w320:dbl)
              n203 = global write "Robot Global Data.vi" "Starting time"(w320) -> ()
              n204 = global write "Robot Global Data.vi" "State Machine"(T20."Firing" ("State Machine")) -> ()
              n205 = call <vilib>:"WPI_DriverStationLCDWrite User Message.vi"("line text"="FIRE BTNS PRESSED", "line"=WPI_DriverStationLCDLCDLine."User - Line 3", "clear line before write (T)"=TRUE) -> ()  [unwired: 12 in, 1 out]
            }
            frame 1 {
              n206 = call <vilib>:"WPI_DriverStationLCDWrite User Message.vi"("line text"="CANNOT FIRE: Vac On", "line"=WPI_DriverStationLCDLCDLine."User - Line 3", "clear line before write (T)"=TRUE) -> ()  [unwired: 12 in, 1 out]
            }
          }
        }
      }
      n207 = global write "Robot Global Data.vi" "Current State Name"(w310) -> ()
      n208 = global write "Robot Global Data.vi" "Waiting For Event"("Both Btn1s" ("Waiting For Event")) -> ()
    }
    frame "Firing" {
      w347 = "Firing" ("line text")
      # "NEED THIS??"
      # "Turn Off Vacuum"
      # "Run Trigger motor forward until hit forward limit, or when watchdog expires"
      n209 = global read "Robot Global Data.vi" "Starting time"() -> (w334:dbl)
      n210 = global read "Robot Global Data.vi" "Fire Limit F"() -> (w332:bool)
      n211 = call <vilib>:"SD Write String.vi"("Table Prefix"=w347, "Name"="State Machine State Name") -> ()  [unwired: 8 in, 2 out]
      n212 = Greater Or Equal?(x=w333, y=w334) -> (x >= y?=w331:bool)
      n213 = global write "Robot Global Data.vi" "Current State Name"(w347) -> ()
      n214 = Or(x=w332, y=w331) -> (x .or. y?=w330:bool)
      n215 = global write "Robot Global Data.vi" "Waiting For Event"("TF Limit" ("Waiting For Event")) -> ()
      n216 = Select(t=T20."Firing Completed" ("State Machine"), s=w330, f=w348) -> (s? t:f=w328:T20)
      n217 = global write "Robot Global Data.vi" "State Machine"(w328) -> ()
      n218 = Select(t=0.0, s=w330, f=-0.8) -> (s? t:f=w350:dbl)
      n219 = call <vilib>:"WPI_MotorControlRefNum Registry Get.vi"("refnum name"="Fire") -> ("error out"=w355:errorcluster, "MotorControlDevRef"=w354:T13)  [unwired: 9 in]
      n220 = call <vilib>:"WPI_MotorControlSetOutput.vi"("error in (no error)"=w355, "Output"=w350, "MotorControlDevRef"=w354) -> ()  [unwired: 6 in, 3 out]
      n221 = call <vilib>:"WPI_MotorControlRefNum Registry Get.vi"("refnum name"="Vacuum") -> ("error out"=w343:errorcluster, "MotorControlDevRef"=w345:T13)  [unwired: 9 in]
      n222 = call <vilib>:"SD Write Boolean.vi"("Boolean"=TRUE, "Name"="Re-Capture") -> ()  [unwired: 8 in, 2 out]
      n223 = call <vilib>:"SD Write Boolean.vi"("Boolean"=FALSE, "Name"="Ready to Fire") -> ()  [unwired: 8 in, 2 out]
      n224 = call <vilib>:"WPI_MotorControlSetOutput.vi"("error in (no error)"=w343, "Output"=0.0, "MotorControlDevRef"=w345) -> ()  [unwired: 6 in, 3 out]
      n225 = call <vilib>:"SD Write Boolean.vi"("Boolean"=FALSE, "Name"="Vacuum State") -> ()  [unwired: 8 in, 2 out]
    }
    frame "Firing Completed" {
      w361 = "Firing Completed" ("line text")
      # "Set delay timer to give give arm time to complete movement before re-engaging gearbox"
      # "Turn off Trigger motor"
      n226 = Add(x=1.5 ("Starting time"), y=w357) -> (x+y=w358:dbl)
      n227 = global write "Robot Global Data.vi" "Starting time"(w358) -> ()
      n228 = call <vilib>:"WPI_MotorControlRefNum Registry Get.vi"("refnum name"="Fire") -> ("error out"=w366:errorcluster, "MotorControlDevRef"=w365:T13)  [unwired: 9 in]
      n229 = call <vilib>:"WPI_MotorControlSetOutput.vi"("error in (no error)"=w366, "Output"=0.0, "MotorControlDevRef"=w365) -> ()  [unwired: 6 in, 3 out]
      n230 = call <vilib>:"SD Write String.vi"("Table Prefix"=w361, "Name"="State Machine State Name") -> ()  [unwired: 8 in, 2 out]
      n231 = global write "Robot Global Data.vi" "State Machine"(T20."Reengage Gearbox" ("State Machine")) -> ()
      n232 = global write "Robot Global Data.vi" "Current State Name"(w361) -> ()
      n233 = global write "Robot Global Data.vi" "Waiting For Event"("Auto" ("Waiting For Event")) -> ()
    }
    frame "Reengage Gearbox" {
      w372 = "Reengage Gearbox" ("line text")
      n234 = global read "Robot Global Data.vi" "Starting time"() -> (w370:dbl)
      n235 = Greater Or Equal?(x=w368, y=w370) -> (x >= y?=w369:bool)
      n236 = call <vilib>:"SD Write String.vi"("Table Prefix"=w372, "Name"="State Machine State Name") -> ()  [unwired: 8 in, 2 out]
      n237 = case shown="True" w369 {
        tunnel: w368 -> [_ w375]
        frame False {
        }
        frame True {
          # "Re-engage Gearbox by running clutch motor in reverse"
          n238 = global write "Robot Global Data.vi" "State Machine"(T20."Reset Delay" ("State Machine")) -> ()
          n239 = call <vilib>:"WPI_ServoRefNum Registry Get.vi"("refnum name"="Gear Box Servo") -> ("error out"=w379:errorcluster, "ServoDeviceRef"=w380:T23)  [unwired: 9 in]
          n240 = Add(x=w375, y=1.0) -> (x+y=w376:dbl)
          n241 = call <vilib>:"WPI_ServoSetAngle.vi"("error in (no error)"=w379, "Angle"=120, "ServoDeviceRef"=w380) -> ()  [unwired: 7 in, 2 out]
          n242 = global write "Robot Global Data.vi" "Starting time"(w376) -> ()
        }
      }
      n243 = global write "Robot Global Data.vi" "Current State Name"(w372) -> ()
      n244 = global write "Robot Global Data.vi" "Waiting For Event"("Timer" ("Waiting For Event")) -> ()
    }
  }
  n245 = case shown="True" w76 {
    tunnel: [w383 w385] -> w2
    tunnel: w1 -> [_ w384]
    frame False {
      n246 = global read "Robot Global Data.vi" "VacuumLatched button"() -> (w383:dbl)
    }
    frame True {
      n247 = global read "Robot Global Data.vi" "VacuumLatched button"() -> (w389:dbl)
      n248 = Less Or Equal To 0?(x=w389) -> (x <= 0?=w386:bool)
      n249 = call <vilib>:"SD Write Boolean.vi"("Boolean"=w386, "Name"="Vacuum State") -> ()  [unwired: 8 in, 2 out]
      n250 = Select(t=1.0 ("Numeric"), s=w386, f=-1.0) -> (s? t:f=w385:dbl)
      n251 = global write "Robot Global Data.vi" "VacuumLatched button"(w385) -> ()
      n252 = global write "Robot Global Data.vi" "Starting time 2"(w384) -> ()
    }
  }
  n253 = global read "Robot Global Data.vi" "Gear Box button"() -> (w55:bool)
  n254 = global write "Robot Global Data.vi" "Vacuum Button"(w80) -> ()
  n255 = Not(x=w55) -> (.not. x?=w56:bool)
  n256 = And(x=w19, y=w56) -> (x .and. y?=w14:bool)
  n257 = global write "Robot Global Data.vi" "Gear Box button"(w19) -> ()
  n258 = case shown="True" w14 {
    frame False {
    }
    frame True {
      n259 = global read "Robot Global Data.vi" "Gear Box Servo Value"() -> (w398:dbl)
      n260 = Less Or Equal To 0?(x=w398) -> (x <= 0?=w395:bool)
      n261 = call <vilib>:"WPI_ServoRefNum Registry Get.vi"("refnum name"="Gear Box Servo") -> ("error out"=w391:errorcluster, "ServoDeviceRef"=w392:T23)  [unwired: 9 in]
      n262 = Select(t=120.0 ("Numeric"), s=w395, f=0.0) -> (s? t:f=w393:dbl)
      n263 = global write "Robot Global Data.vi" "Gear Box Servo Value"(w393) -> ()
      n264 = call <vilib>:"WPI_ServoSetAngle.vi"("error in (no error)"=w391, "Angle"=w393, "ServoDeviceRef"=w392) -> ()  [unwired: 7 in, 2 out]
    }
  }
  n265 = case shown="-1, Default" w2 {
    tunnel: w2 -> [w400 w412 w416]
    tunnel: w1 -> [w405 _ _]
    frame -1, Default {
      n266 = global read "Robot Global Data.vi" "Starting time 2"() -> (w407:dbl)
      n267 = call <vilib>:"WPI_MotorControlRefNum Registry Get.vi"("refnum name"="Vacuum") -> ("error out"=w401:errorcluster, "MotorControlDevRef"=w402:T13)  [unwired: 9 in]
      n268 = call <vilib>:"WPI_MotorControlSetOutput.vi"("error in (no error)"=w401, "Output"=w400, "MotorControlDevRef"=w402) -> ()  [unwired: 6 in, 3 out]
      n269 = Add(x=w407, y=0.25) -> (x+y=w406:dbl)
      n270 = Greater Or Equal?(x=w405, y=w406) -> (x >= y?=w404:bool)
      n271 = Select(t=0.0, s=w404, f=w400) -> (s? t:f=w403:dbl)
      n272 = global write "Robot Global Data.vi" "VacuumLatched button"(w403) -> ()
    }
    frame 0 {
      n273 = call <vilib>:"WPI_MotorControlRefNum Registry Get.vi"("refnum name"="Vacuum") -> ("error out"=w410:errorcluster, "MotorControlDevRef"=w411:T13)  [unwired: 9 in]
      n274 = call <vilib>:"WPI_MotorControlSetOutput.vi"("error in (no error)"=w410, "Output"=w412, "MotorControlDevRef"=w411) -> ()  [unwired: 6 in, 3 out]
    }
    frame 1 {
      n275 = call <vilib>:"WPI_MotorControlRefNum Registry Get.vi"("refnum name"="Vacuum") -> ("error out"=w414:errorcluster, "MotorControlDevRef"=w415:T13)  [unwired: 9 in]
      n276 = call <vilib>:"WPI_MotorControlSetOutput.vi"("error in (no error)"=w414, "Output"=w416, "MotorControlDevRef"=w415) -> ()  [unwired: 6 in, 3 out]
    }
  }
  n277 = disable-structure shown="Disabled" {
    frame Disabled {
      n278 = call <vilib>:"WPI_AnalogChannelRefNum Registry Get.vi"("refnum name"="Potentiometer") -> ("error out"=w424:errorcluster, "AIDeviceRef"=w423:T24)  [unwired: 9 in]
      n279 = call <vilib>:"WPI_AnalogChannelGetAverageVoltage.vi"("error in (no error)"=w424, "AIDeviceRef"=w423) -> ("Voltage"=w419:dbl)  [unwired: 7 in, 2 out]
      n280 = Multiply(x=w419, y=45.0) -> (x*y=w418:dbl)
      n281 = call <vilib>:"SD Write Number.vi"("Numeric"=w418, "Name"="Pot") -> ()  [unwired: 8 in, 2 out]
    }
    frame Enabled {
    }
  }
  n282 = global read "Robot Global Data.vi" "Arm Limit B"() -> (w33:bool)
  n283 = global read "Robot Global Data.vi" "Arm Limit F"() -> (w34:bool)
  n284 = global read "Robot Global Data.vi" "Defender"() -> (w17:bool)
  n285 = global read "Robot Global Data.vi" "VacuumLatched button"() -> (w67:dbl)
  n286 = Not(x=w17) -> (.not. x?=w16:bool)
  n287 = global write "Robot Global Data.vi" "Defender"(w18) -> ()
  n288 = Or(x=w34, y=w33) -> (x .or. y?=w84:bool)
  n289 = case shown="True" w84 {
    tunnel: w77 -> [w425 w430]
    tunnel: [w425 w428] -> w75
    frame False {
    }
    frame True {
      n290 = global read "Robot Global Data.vi" "Arm Limit B"() -> (w427:bool)
      n291 = case shown="True" w427 {
        tunnel: w430 -> [w440 w446]
        tunnel: [w440 w448] -> w429
        frame False {
        }
        frame True {
          n292 = Greater?(x=w446, y=0.0) -> (0:w444:bool)
          n293 = Select(t=w446, s=w444, f=0.0) -> (s? t:f=w448:dbl)
          n294 = call <vilib>:"WPI_DriverStationLCDWrite User Message.vi"("line text"="Back Arm Limit", "line"=WPI_DriverStationLCDLCDLine."User - Line 5", "clear line before write (T)"=TRUE) -> ()  [unwired: 12 in, 1 out]
        }
      }
      n295 = global read "Robot Global Data.vi" "Arm Limit F"() -> (w426:bool)
      n296 = case shown="True" w426 {
        tunnel: w429 -> [w431 w437]
        tunnel: [w431 w439] -> w428
        frame False {
        }
        frame True {
          n297 = Less?(x=w437, y=0.0) -> (x < y?=w435:bool)
          n298 = Select(t=w437, s=w435, f=0.0) -> (s? t:f=w439:dbl)
          n299 = call <vilib>:"WPI_DriverStationLCDWrite User Message.vi"("line text"="Forward Arm Limit", "line"=WPI_DriverStationLCDLCDLine."User - Line 5", "clear line before write (T)"=TRUE) -> ()  [unwired: 12 in, 1 out]
        }
      }
    }
  }
  n300 = And(x=w18, y=w16) -> (x .and. y?=w15:bool)
  n301 = call <vilib>:"WPI_ServoRefNum Registry Get.vi"("refnum name"="Gear Box Servo") -> ("error out"=w3:errorcluster, "ServoDeviceRef"=w4:T23)  [unwired: 9 in]
  n302 = call <vilib>:"WPI_ServoGetAngle.vi"("ServoDeviceRef"=w4, "error in (no error)"=w3) -> ("Angle"=w6:u16)  [unwired: 6 in, 2 out]
  n303 = Greater Than 0?(x=w67) -> (x > 0?=w68:bool)
  n304 = Greater Than 0?(x=w6) -> (x > 0?=w7:bool)
  n305 = Select(t="Vac Is On   ", s=w68, f="Vac Is Off    ") -> (s? t:f=w74:string)
  n306 = call <vilib>:"WPI_DriverStationLCDWrite User Message.vi"("line text"=w74, "line"=WPI_DriverStationLCDLCDLine."User - Line 2", "starting column"=i8 1, "clear line before write (T)"=FALSE) -> ()  [unwired: 11 in, 1 out]
  n307 = Select(t="GearBox Engaged       ", s=w7, f="GearBox Disengaged") -> (s? t:f=w13:string)
  n308 = call <vilib>:"WPI_DriverStationLCDWrite User Message.vi"("line text"=w13, "line"=WPI_DriverStationLCDLCDLine."User - Line 5", "starting column"=i8 1, "clear line before write (T)"=FALSE) -> ()  [unwired: 11 in, 1 out]
  n309 = case shown="True" w15 {
    frame False {
    }
    frame True {
      n310 = global read "Robot Global Data.vi" "Defender State"() -> (w451:dbl)
      n311 = case shown="3" w451 {
        tunnel: [1.0 ("Defender State") 2.0 ("Defender State") 3.0 ("Defender State") 0.0 ("Defender State")] -> w450
        tunnel: [1.0 ("Numeric") 0.0 ("Numeric") -1.0 ("Numeric") 0.0 ("Numeric")] -> w449
        frame 0, Default {
        }
        frame 1 {
        }
        frame 2 {
        }
        frame 3 {
        }
      }
      n312 = call <vilib>:"WPI_MotorControlRefNum Registry Get.vi"("refnum name"="Defender") -> ("error out"=w452:errorcluster, "MotorControlDevRef"=w453:T13)  [unwired: 9 in]
      n313 = call <vilib>:"WPI_MotorControlSetOutput.vi"("error in (no error)"=w452, "Output"=w449, "MotorControlDevRef"=w453) -> ()  [unwired: 6 in, 3 out]
      n314 = global write "Robot Global Data.vi" "Defender State"(w450) -> ()
    }
  }
  n315 = call <vilib>:"WPI_MotorControlRefNum Registry Get.vi"("refnum name"="Arm") -> ("MotorControlDevRef"=w86:T13)  [unwired: 9 in, 1 out]
  n316 = call <vilib>:"WPI_MotorControlSetOutput.vi"("Output"=w75, "MotorControlDevRef"=w86) -> ()  [unwired: 7 in, 3 out]
  n317 = disable-structure shown="Disabled" {
    frame Disabled {
      n318 = call <vilib>:"WPI_RelayRefNum Registry Get.vi"("refnum name"="fire") -> ("error out"=w464:errorcluster, "RelayDevRef"=w465:T27)  [unwired: 9 in]
      n319 = call <vilib>:"WPI_RelaySet.vi"("error in (no error)"=w464, "RelayDevRef"=w465) -> ()  [unwired: 8 in, 2 out]
    }
    frame Enabled {
    }
  }
